vi "Test_ConfigFile_ReadEnum.vi"() -> ()   [LabVIEW 2020]
uses:
  <vilib>/Utility/config.llb/NI_LVConfig.lvlib
panel:
  out "error out":errorcluster
  out "SelectSomething":enum16{"Item1", "Item2", "Item3", "Test Item"}(ring)
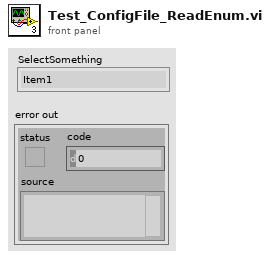
[diagram p1: front panel]
types:
  T1 = typedef "NI_LVConfig.lvlib/Config Data RefNum.ctl" = refnum<k1>
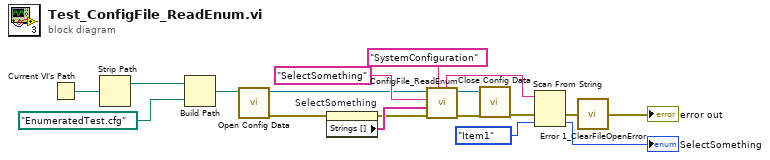
[diagram p0: block diagram]
diagram:
  n1 = Current VI's Path() -> (path=w4:path)
  n2 = Strip Path(path=w4) -> (stripped path=w3:path)  [unwired: 1 out]
  n3 = Build Path(base path=w3, name or relative path=path "EnumeratedTest.cfg" ("configuration file path")) -> (appended path=w1:path)
  n4 = call <vilib>:"Open Config Data.vi"("configuration file path"=w1) -> ("error out"=w16:errorcluster, "refnum"=w12:T1)  [unwired: 8 in, 1 out]
  n5 = property on="SelectSomething" class="Enum (strict)"(error in=w16) -> (error out=w15:errorcluster, "Strings []"=w18:string[])  [unwired: 1 in, 1 out]
  n6 = call "ConfigFile_ReadEnum.vi"("CFG.SectionName"="SystemConfiguration" ("sectionName"), "error in (no error)"=w15, "Enum.Strings[]"=w18, "Enum.Label"="SelectSomething" ("configItemName"), "ConfigFileRef"=w12) -> ("error out"=w14:errorcluster, "ConfigFileRef.DUP"=w13:T1, "EnumSelection.Out"=w5:string)  [unwired: 3 in, 1 out]
  n7 = call <vilib>:"Close Config Data.vi"("error in (no error)"=w14, "refnum"=w13) -> ("error out"=w8:errorcluster)  [unwired: 8 in, 1 out]
  n8 = Scan From String(input string=w5, error in=w8, default 1=enum16{"Item1", "Item2", "Item3", "Test Item"}."Item1" ("SelectSomething")) -> (error out=w7:errorcluster, output 1=→"SelectSomething":enum16{"Item1", "Item2", "Item3", "Test Item"})  [unwired: 2 in, 2 out]
  n9 = call "Error 1_ClearFileOpenError.vi"("error in"=w7) -> ("error out"=→"error out":errorcluster)  [unwired: 4 in]
